vi "RADI Peak Senzora.vi"() -> ()   [LabVIEW 2017]
uses:
  Grafik.ctl
  <vilib>/Waveform/WDTOps.llb/WDT Index Channel DBL.vi
panel:
  in  "Tab Control":enum32{"FRONT", "LIVE DATA", "Podesavanja"}(tab)
  in  "Brzina App":i16(slide)=1900 caption="Speed" min=500 max=1900 step=100 scale=500.0..1900.0
  out "3":bool
  out "2":bool
  out "1":bool
  out "Waveform Graph":T1
  out "?":dbl format="%#5_3g"
  out "Inteziteti ACC 1":waveform(dbl)(graph)
  out "Inteziteti ACC 2":waveform(dbl)(graph)
  out "Inteziteti ACC 3":waveform(dbl)(graph)
  out "TRENUTNI SIGNALI":dynamicdata(graph) caption="TRENUTNI SIGNALI !!!!"
  out "GORE":bool
  in  "File Name":string="TEST"
  in  "Ponavljanja":i32=40
  out "ULAZ ANN":dbl[](array[numeric])
  out "Niz":dbl[](array[numeric])
  out "Matrica":dbl[][](array[numeric])
  out "error out":errorcluster
  out "BROJ":dbl
  out "SREDINA":bool
  out "DOLE":bool
  out "sum":dbl
  out "Sekvenca":dbl[](array[numeric])
  in  "Kombinacije":string(combo)="Combinations_1 - Srpski_Brojevi"
  out "Iter":i32
  out "SCORE":dbl
  in  "VREME 100mS":i16(knob)=1900 min=500 max=19000 step=100 scale=500.0..1900.0
  # "'Gore 1, Sredina 2, Dole 4, Miruje 8'"
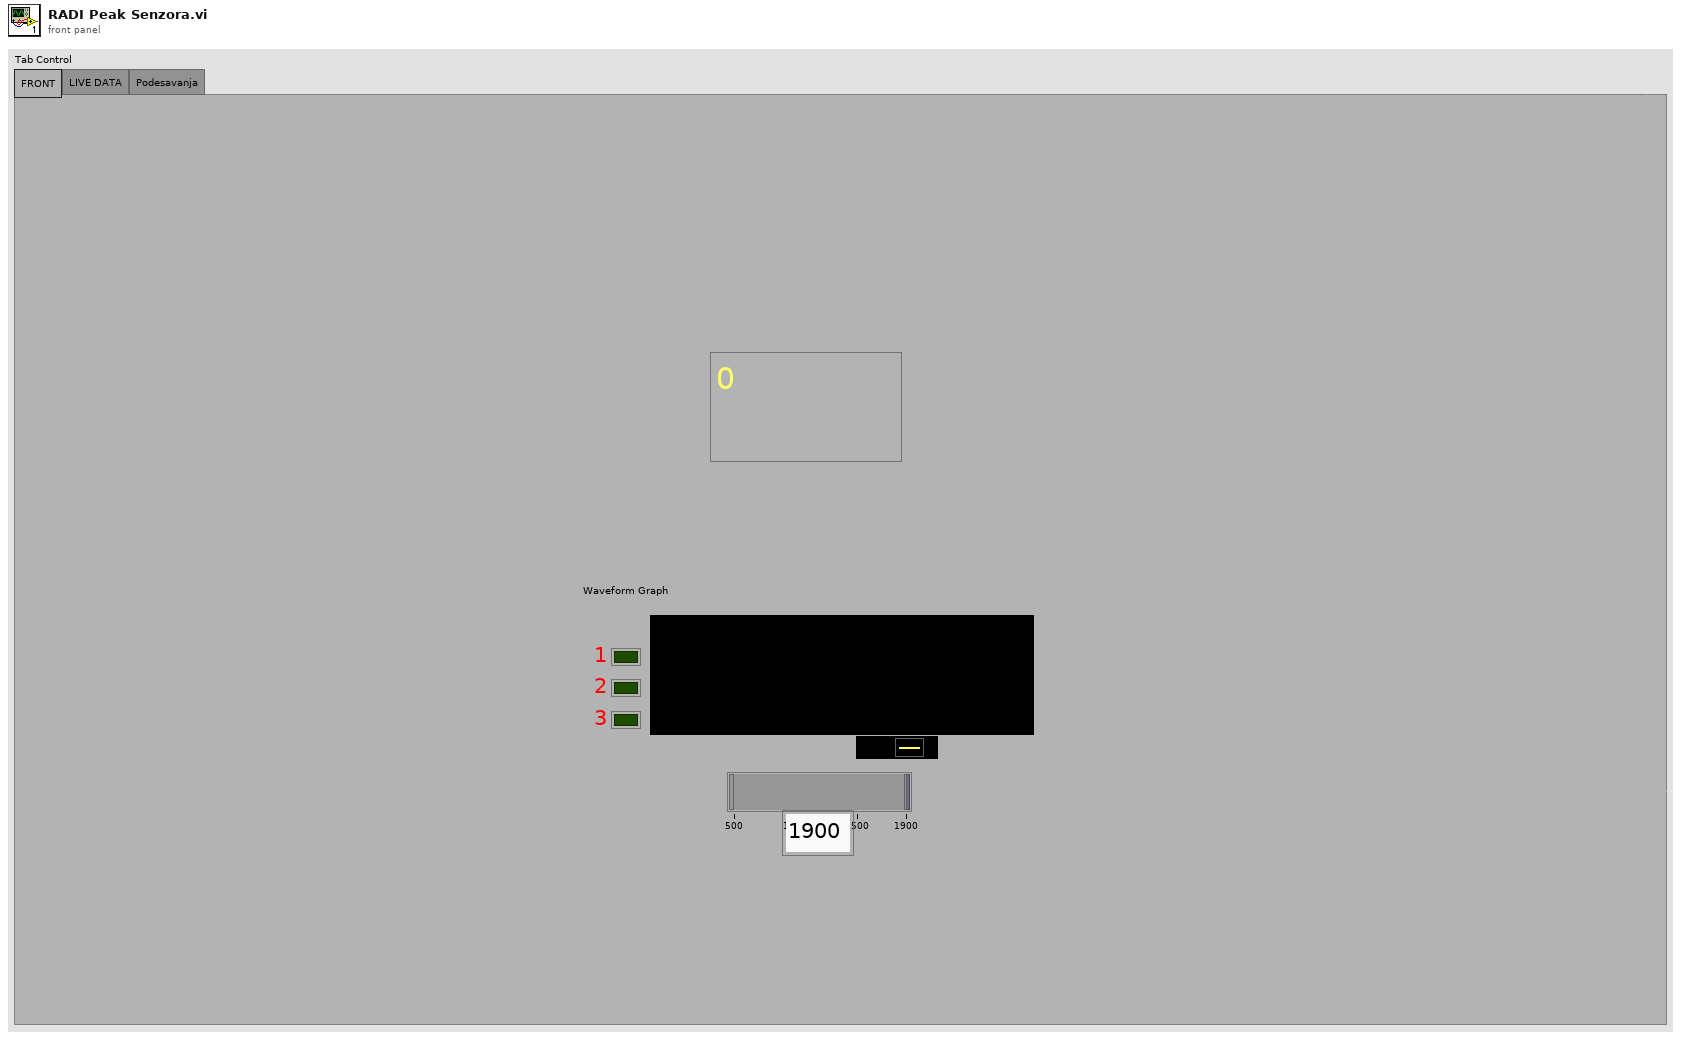
[diagram p1: front panel]
types:
  T1 = typedef "Grafik.ctl" = dynamicdata
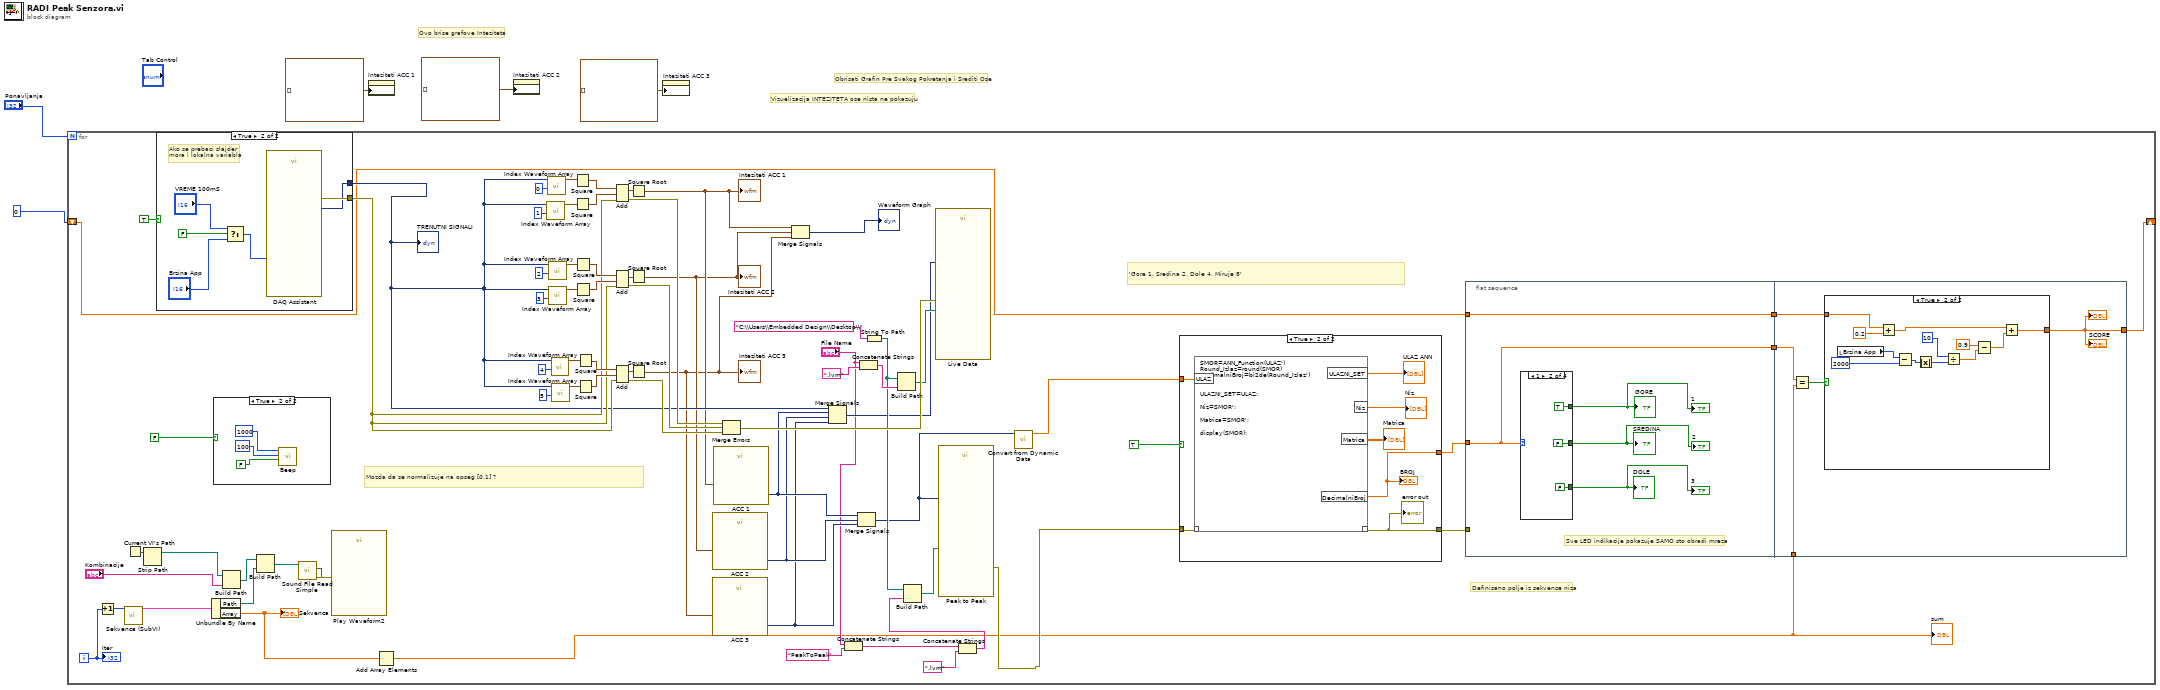
[diagram p0: block diagram]
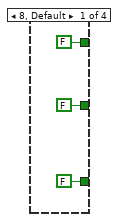
[diagram p3: hidden frame]
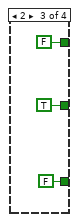
[diagram p4: hidden frame]
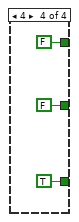
[diagram p5: hidden frame]
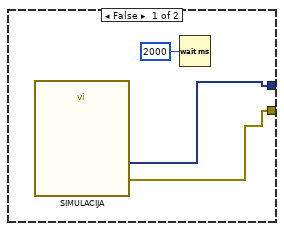
[diagram p7: hidden frame]
diagram:
  # "Ovo brise grafove Inteziteta"
  # "Obrisati Grafin Pre Svakog Pokretanja i Srediti Ose"
  # "Vizuelizacija INTEZITETA ose nista ne pokazuju"
  n1 = for {
    N: "Ponavljanja" -> [_]
    shift-right: [w6] -> _
    shift-left: 0 -> [w16]
    i -> [w18]
    # "Definisano polje iz sekvence niza"
    # "'Gore 1, Sredina 2, Dole 4, Miruje 8'"
    # "Mozda da se normalizuje na opseg [0,1] ?"
    n2 = Increment(x=w18) -> (x+1=w19:i32)
    n3 = call "Sekvenca (SubVI).vi"("Ulaz"=w19) -> ("Cluster 41"=w21:cluster{"Path":path, "Array":dbl[]})  [unwired: 9 in, 1 out]
    n4 = Current VI's Path() -> (path=w27:path)
    n5 = Strip Path(path=w27) -> (stripped path=w24:path)  [unwired: 1 out]
    n6 = case shown="True" TRUE {
      tunnel: [w116 w123] -> w50
      tunnel: [w117 w122] -> w31
      frame False {
        n7 = call "SIMULACIJA"() -> ("data"=w117:dynamicdata, "error out"=w116:errorcluster)  [unwired: 17 in, 1 out]
        n8 = Wait (ms)(milliseconds to wait=u32 2000) -> ()  [unwired: 1 out]
      }
      frame True {
        # "Ako se prebaci slajder\nmora i lokalna variabla"
        n9 = Select(t="VREME 100mS", s=FALSE, f="Brzina App") -> (s? t:f=w119:i16)
        n10 = call "DAQ Assistant"("number of samples"=w119) -> ("data"=w122:dynamicdata, "error out"=w123:errorcluster)  [unwired: 15 in, 2 out]
      }
    }
    "TRENUTNI SIGNALI" <- w31
    n11 = Unbundle By Name(w21) -> ("Path"=w22:path, "Array"=w17:dbl[])
    "Sekvenca" <- w17
    n12 = case shown="True" FALSE {
      frame False {
      }
      frame True {
        n13 = call <vilib>:"Beep.vi"("use system alert? (T)"=FALSE, "duration (msec)"=u32 100, "frequency (Hz)"=u32 1000) -> ()  [unwired: 9 in]
      }
    }
    n14 = Build Path(base path=w24, name or relative path="Kombinacije") -> (appended path=w26:path)
    n15 = Build Path(base path=w26, name or relative path=w22) -> (appended path=w25:path)
    n16 = call <vilib>:"Sound File Read Simple.vi"("path"=w25) -> ("error out"=w28:errorcluster, "data"=w23:waveform(dbl)[])  [unwired: 7 in, 2 out]
    n17 = call "Play Waveform2"("Data"=w23, "error in"=w28) -> ()  [unwired: 17 in, 1 out]
    n18 = Add Array Elements(numeric array=w17) -> (sum=w7:dbl)
    "sum" <- w7
    n19 = call-poly <vilib>:"Index Waveform Array.vi"("index"=1, "waveform array"=w31) -> ("waveform"=w64:waveform(dbl))  [unwired: 8 in, 1 out]
    n20 = call-poly <vilib>:"Index Waveform Array.vi"("index"=0, "waveform array"=w31) -> ("waveform"=w65:waveform(dbl))  [unwired: 8 in, 1 out]
    n21 = call-poly <vilib>:"Index Waveform Array.vi"("index"=2, "waveform array"=w31) -> ("waveform"=w63:waveform(dbl))  [unwired: 8 in, 1 out]
    n22 = call-poly <vilib>:"Index Waveform Array.vi"("index"=3, "waveform array"=w31) -> ("waveform"=w62:waveform(dbl))  [unwired: 8 in, 1 out]
    n23 = call-poly <vilib>:"Index Waveform Array.vi"("index"=4, "waveform array"=w31) -> ("waveform"=w61:waveform(dbl))  [unwired: 8 in, 1 out]
    n24 = call-poly <vilib>:"Index Waveform Array.vi"("index"=5, "waveform array"=w31) -> ("waveform"=w60:waveform(dbl))  [unwired: 8 in, 1 out]
    n25 = Square(x=w65) -> (x^2=w59:waveform(dbl))
    n26 = Square(x=w64) -> (x^2=w58:waveform(dbl))
    n27 = Square(x=w63) -> (x^2=w57:waveform(dbl))
    n28 = Square(x=w62) -> (x^2=w56:waveform(dbl))
    n29 = Square(x=w61) -> (x^2=w55:waveform(dbl))
    n30 = Square(x=w60) -> (x^2=w54:waveform(dbl))
    n31 = Add(1:w58, 2:w59, 4:w50) -> (0:w53:waveform(dbl), 3:w49:errorcluster)
    n32 = Add(1:w56, 2:w57, 4:w50) -> (0:w52:waveform(dbl), 3:w48:errorcluster)
    n33 = Add(1:w54, 2:w55, 4:w50) -> (0:w51:waveform(dbl), 3:w47:errorcluster)
    n34 = Square Root(x=w53) -> (sqrt(x)=w15:waveform(dbl))
    "Inteziteti ACC 1" <- w15
    n35 = Square Root(x=w52) -> (sqrt(x)=w14:waveform(dbl))
    "Inteziteti ACC 2" <- w14
    n36 = Square Root(x=w51) -> (sqrt(x)=w13:waveform(dbl))
    "Inteziteti ACC 3" <- w13
    n37 = call "ACC 3"("Signals"=w13) -> ("Peak to Peak"=w40:dynamicdata)  [unwired: 13 in, 1 out]
    n38 = call "ACC 2"("Signals"=w14) -> ("Peak to Peak"=w41:dynamicdata)  [unwired: 13 in, 1 out]
    n39 = call "ACC 1"("Signals"=w15) -> ("Peak to Peak"=w42:dynamicdata)  [unwired: 13 in, 1 out]
    n40 = Merge Errors(w49, w48, w47) -> (w76:errorcluster)
    n41 = Merge Signals(w15, w14, w13) -> (→"Waveform Graph":dynamicdata)
    n42 = Merge Signals(w31, w42, w41, w40) -> (w43:dynamicdata)
    n43 = Concatenate Strings("File Name", "PeakToPeak" ("File Name 2")) -> (w37:string)
    n44 = Merge Signals(w42, w41, w40) -> (w34:dynamicdata)
    n45 = Concatenate Strings("File Name", ".lvm" ("name or relative path")) -> (w72:string)
    n46 = String To Path(string="C:\\Users\\Embedded Design\\Desktop\\") -> (path=w44:path)
    n47 = Build Path(base path=w44, name or relative path=w72) -> (appended path=w75:path)
    n48 = call "Live Data"("Signals"=w43, "error in (no error)"=w76, "Filename"=w75) -> ()  [unwired: 14 in, 3 out]
    n49 = Concatenate Strings(w37, ".lvm" ("name or relative path")) -> (w46:string)
    n50 = Build Path(base path=w44, name or relative path=w46) -> (appended path=w45:path)
    n51 = call "Peak to Peak"("Signals"=w34, "Filename"=w45) -> ("error out"=w35:errorcluster)  [unwired: 15 in, 2 out]
    n52 = call "Convert from Dynamic Data"("Dynamic Data Type"=w34) -> ("Array"=w33:dbl[])  [unwired: 3 in]
    n53 = case shown="True" TRUE {
      tunnel: w35 -> [w124 w131]
      tunnel: w33 -> [_ w130]
      tunnel: [w124 w126] -> w29
      tunnel: [_ w125] -> w11
      frame False {
      }
      frame True {
        n54 = script code="SMOR=ANN_Function(ULAZ')\nRound_Izlaz=round(SMOR)\nDecimalniBroj=bi2de(Round_Izlaz')\n\n\nULAZNI_SET=ULAZ;\n\nNiz=SMOR';\n\nMatrica=SMOR';\n\ndisplay(SMOR);"("??"=w131, "ULAZ"=w130) -> ("??"=w126:errorcluster, "ULAZNI_SET"=→"ULAZ ANN":dbl[], "Niz"=→"Niz":dbl[], "Matrica"=→"Matrica":dbl[][], "DecimalniBroj"=w125:dbl)
        "error out" <- w126
        "BROJ" <- w125
      }
    }
    n55 = flat-sequence {
      tunnel: w29 -> [_]
      tunnel: w16 -> [w81]
      tunnel: w11 -> [w80]
      tunnel: [w81] -> w9
      tunnel: [w80] -> w8
      tunnel: w9 -> [w100]
      tunnel: w8 -> [w98]
      tunnel: w7 -> [w97]
      tunnel: [w99] -> w6
      frame #0 {
        # "Sve LED indikacije pokazuje SAMO sto obradi mreza"
        n56 = case shown="1" w80 {
          tunnel: [FALSE ("DOLE") FALSE ("DOLE") FALSE ("DOLE") TRUE ("DOLE")] -> w82
          tunnel: [FALSE ("SREDINA") FALSE ("SREDINA") TRUE ("SREDINA") FALSE ("SREDINA")] -> w83
          tunnel: [FALSE ("GORE") TRUE ("GORE") FALSE ("GORE") FALSE ("GORE")] -> w84
          frame 8, Default {
          }
          frame 1 {
          }
          frame 2 {
          }
          frame 4 {
          }
        }
        "GORE" <- w84
        "SREDINA" <- w83
        "DOLE" <- w82
        "1" <- w84
        "2" <- w83
        "3" <- w82
      }
      frame #1 {
        n57 = Equal?(x=w98, y=w97) -> (x = y?=w101:bool)
        n58 = case shown="True" w101 {
          tunnel: w100 -> [w102 w104]
          tunnel: [w102 w103] -> w99
          frame False {
          }
          frame True {
            n59 = local read "Brzina App"() -> (w112:i16)
            n60 = Add(x=w104, y=0.2) -> (x+y=w109:dbl)
            n61 = Subtract(x=w112, y=2000) -> (x-y=w114:i32)
            n62 = Absolute Value(x=w114) -> (abs(x)=w113:i32)
            n63 = Divide(x=10, y=w113) -> (x/y=w111:dbl)
            n64 = Subtract(x=0.9, y=w111) -> (x-y=w110:dbl)
            n65 = Add(x=w109, y=w110) -> (x+y=w103:dbl)
          }
        }
        "SCORE" <- w99
        "?" <- w99
      }
    }
    "Iter" <- w18
  }
  n66 = property on="Inteziteti ACC 1" class="WFChart (strict)"("History Data"=waveform(dbl)[] []) -> ()  [unwired: 2 in, 2 out]
  n67 = property on="Inteziteti ACC 2" class="WFChart (strict)"("History Data"=waveform(dbl)[] []) -> ()  [unwired: 2 in, 2 out]
  n68 = property on="Inteziteti ACC 3" class="WFChart (strict)"("History Data"=waveform(dbl)[] []) -> ()  [unwired: 2 in, 2 out]
